vi "Read Parameters to process.vi"(8 "error in":errorcluster, 11 "MotionModule runtime in":refnum<class "MotionModule runtime.lvclass">) -> (0 "error out":errorcluster, 2 "Parameters to process":T1, 3 "MotionModule runtime out":refnum<class "MotionModule runtime.lvclass">)   [LabVIEW 2017, in "MotionModule runtime.lvclass"]
uses:
  MotionModule runtime.lvclass
  configuration/parameter data indices.ctl
  MotionModule runtime.lvclass/MotionModule runtime.ctl
  configuration/MotionModule configuration.lvclass
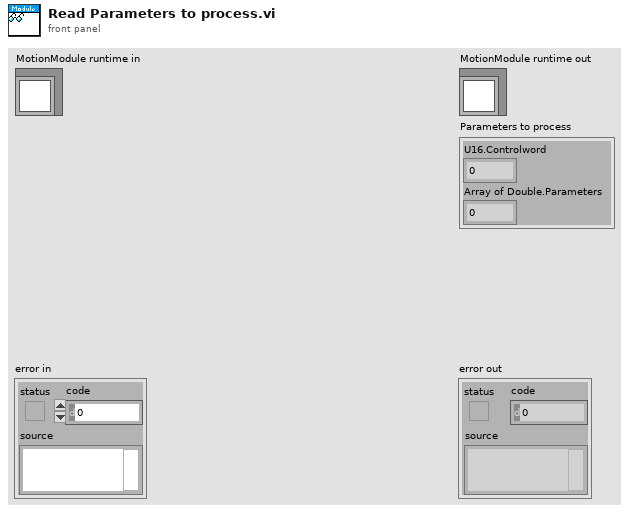
[diagram p1: front panel]
types:
  T1 = typedef "MotionModule configuration.lvclass/parameter data indices.ctl" = cluster{"U16.Controlword":i32, "Array of Double.Parameters":i32}
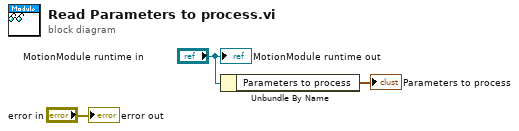
[diagram p0: block diagram]
diagram:
  n1 = Unbundle By Name("MotionModule runtime in") -> ("Parameters to process"=→"Parameters to process":T1)
  "error out" <- "error in"
  "MotionModule runtime out" <- "MotionModule runtime in"
